vi "DEMPSubViewer.vi"() -> ()   [LabVIEW 2022 SP3]
panel:
  out "Channels":T1(array[cluster])
  out "bias":dbl[](array[numeric])
  out "times":dbl[](array[numeric])
  in  "Path":path
  in  "IV Phase":i64=-42
  out "XAxis":dbl[](array[numeric])
  in  "Channel Name":string
  in  "XChannel":bool
  in  "XBias":bool
  in  "XTime":bool
  out "Y Scale":i64
  in  "10 nA":bool
  in  "5nA":bool
  in  "3nA":bool
  in  "1nA":bool
  in  "Y Limits":bool
  out "XY Graph 32":cluster{dbl[], "Data":dbl[]}[](graph)
  out "XY Graph 31":cluster{dbl[], "Data":dbl[]}[](graph)
  out "XY Graph 30":cluster{dbl[], "Data":dbl[]}[](graph)
  out "XY Graph 29":cluster{dbl[], "Data":dbl[]}[](graph)
  out "XY Graph 28":cluster{dbl[], "Data":dbl[]}[](graph)
  out "XY Graph 27":cluster{dbl[], "Data":dbl[]}[](graph)
  out "XY Graph 26":cluster{dbl[], "Data":dbl[]}[](graph)
  out "XY Graph 25":cluster{dbl[], "Data":dbl[]}[](graph)
  out "XY Graph 24":cluster{dbl[], "Data":dbl[]}[](graph)
  out "XY Graph 23":cluster{dbl[], "Data":dbl[]}[](graph)
  out "XY Graph 22":cluster{dbl[], "Data":dbl[]}[](graph)
  out "XY Graph 21":cluster{dbl[], "Data":dbl[]}[](graph)
  out "XY Graph 20":cluster{dbl[], "Data":dbl[]}[](graph)
  out "XY Graph 19":cluster{dbl[], "Data":dbl[]}[](graph)
  out "XY Graph 18":cluster{dbl[], "Data":dbl[]}[](graph)
  out "XY Graph 17":cluster{dbl[], "Data":dbl[]}[](graph)
  out "XY Graph 16":cluster{dbl[], "Data":dbl[]}[](graph)
  out "XY Graph 15":cluster{dbl[], "Data":dbl[]}[](graph)
  out "XY Graph 14":cluster{dbl[], "Data":dbl[]}[](graph)
  out "XY Graph 13":cluster{dbl[], "Data":dbl[]}[](graph)
  out "XY Graph 12":cluster{dbl[], "Data":dbl[]}[](graph)
  out "XY Graph 11":cluster{dbl[], "Data":dbl[]}[](graph)
  out "XY Graph 10":cluster{dbl[], "Data":dbl[]}[](graph)
  out "XY Graph 9":cluster{dbl[], "Data":dbl[]}[](graph)
  out "XY Graph 3":cluster{dbl[], "Data":dbl[]}[](graph)
  out "XY Graph 8":cluster{dbl[], "Data":dbl[]}[](graph)
  out "XY Graph 7":cluster{dbl[], "Data":dbl[]}[](graph)
  out "XY Graph 6":cluster{dbl[], "Data":dbl[]}[](graph)
  out "XY Graph 5":cluster{dbl[], "Data":dbl[]}[](graph)
  out "XY Graph 4":cluster{dbl[], "Data":dbl[]}[](graph)
  out "XY Graph 2":cluster{dbl[], "Data":dbl[]}[](graph)
  out "XY Graph 1":cluster{dbl[], "Data":dbl[]}[](graph)
  in  "stop":bool
  # "X Axis"
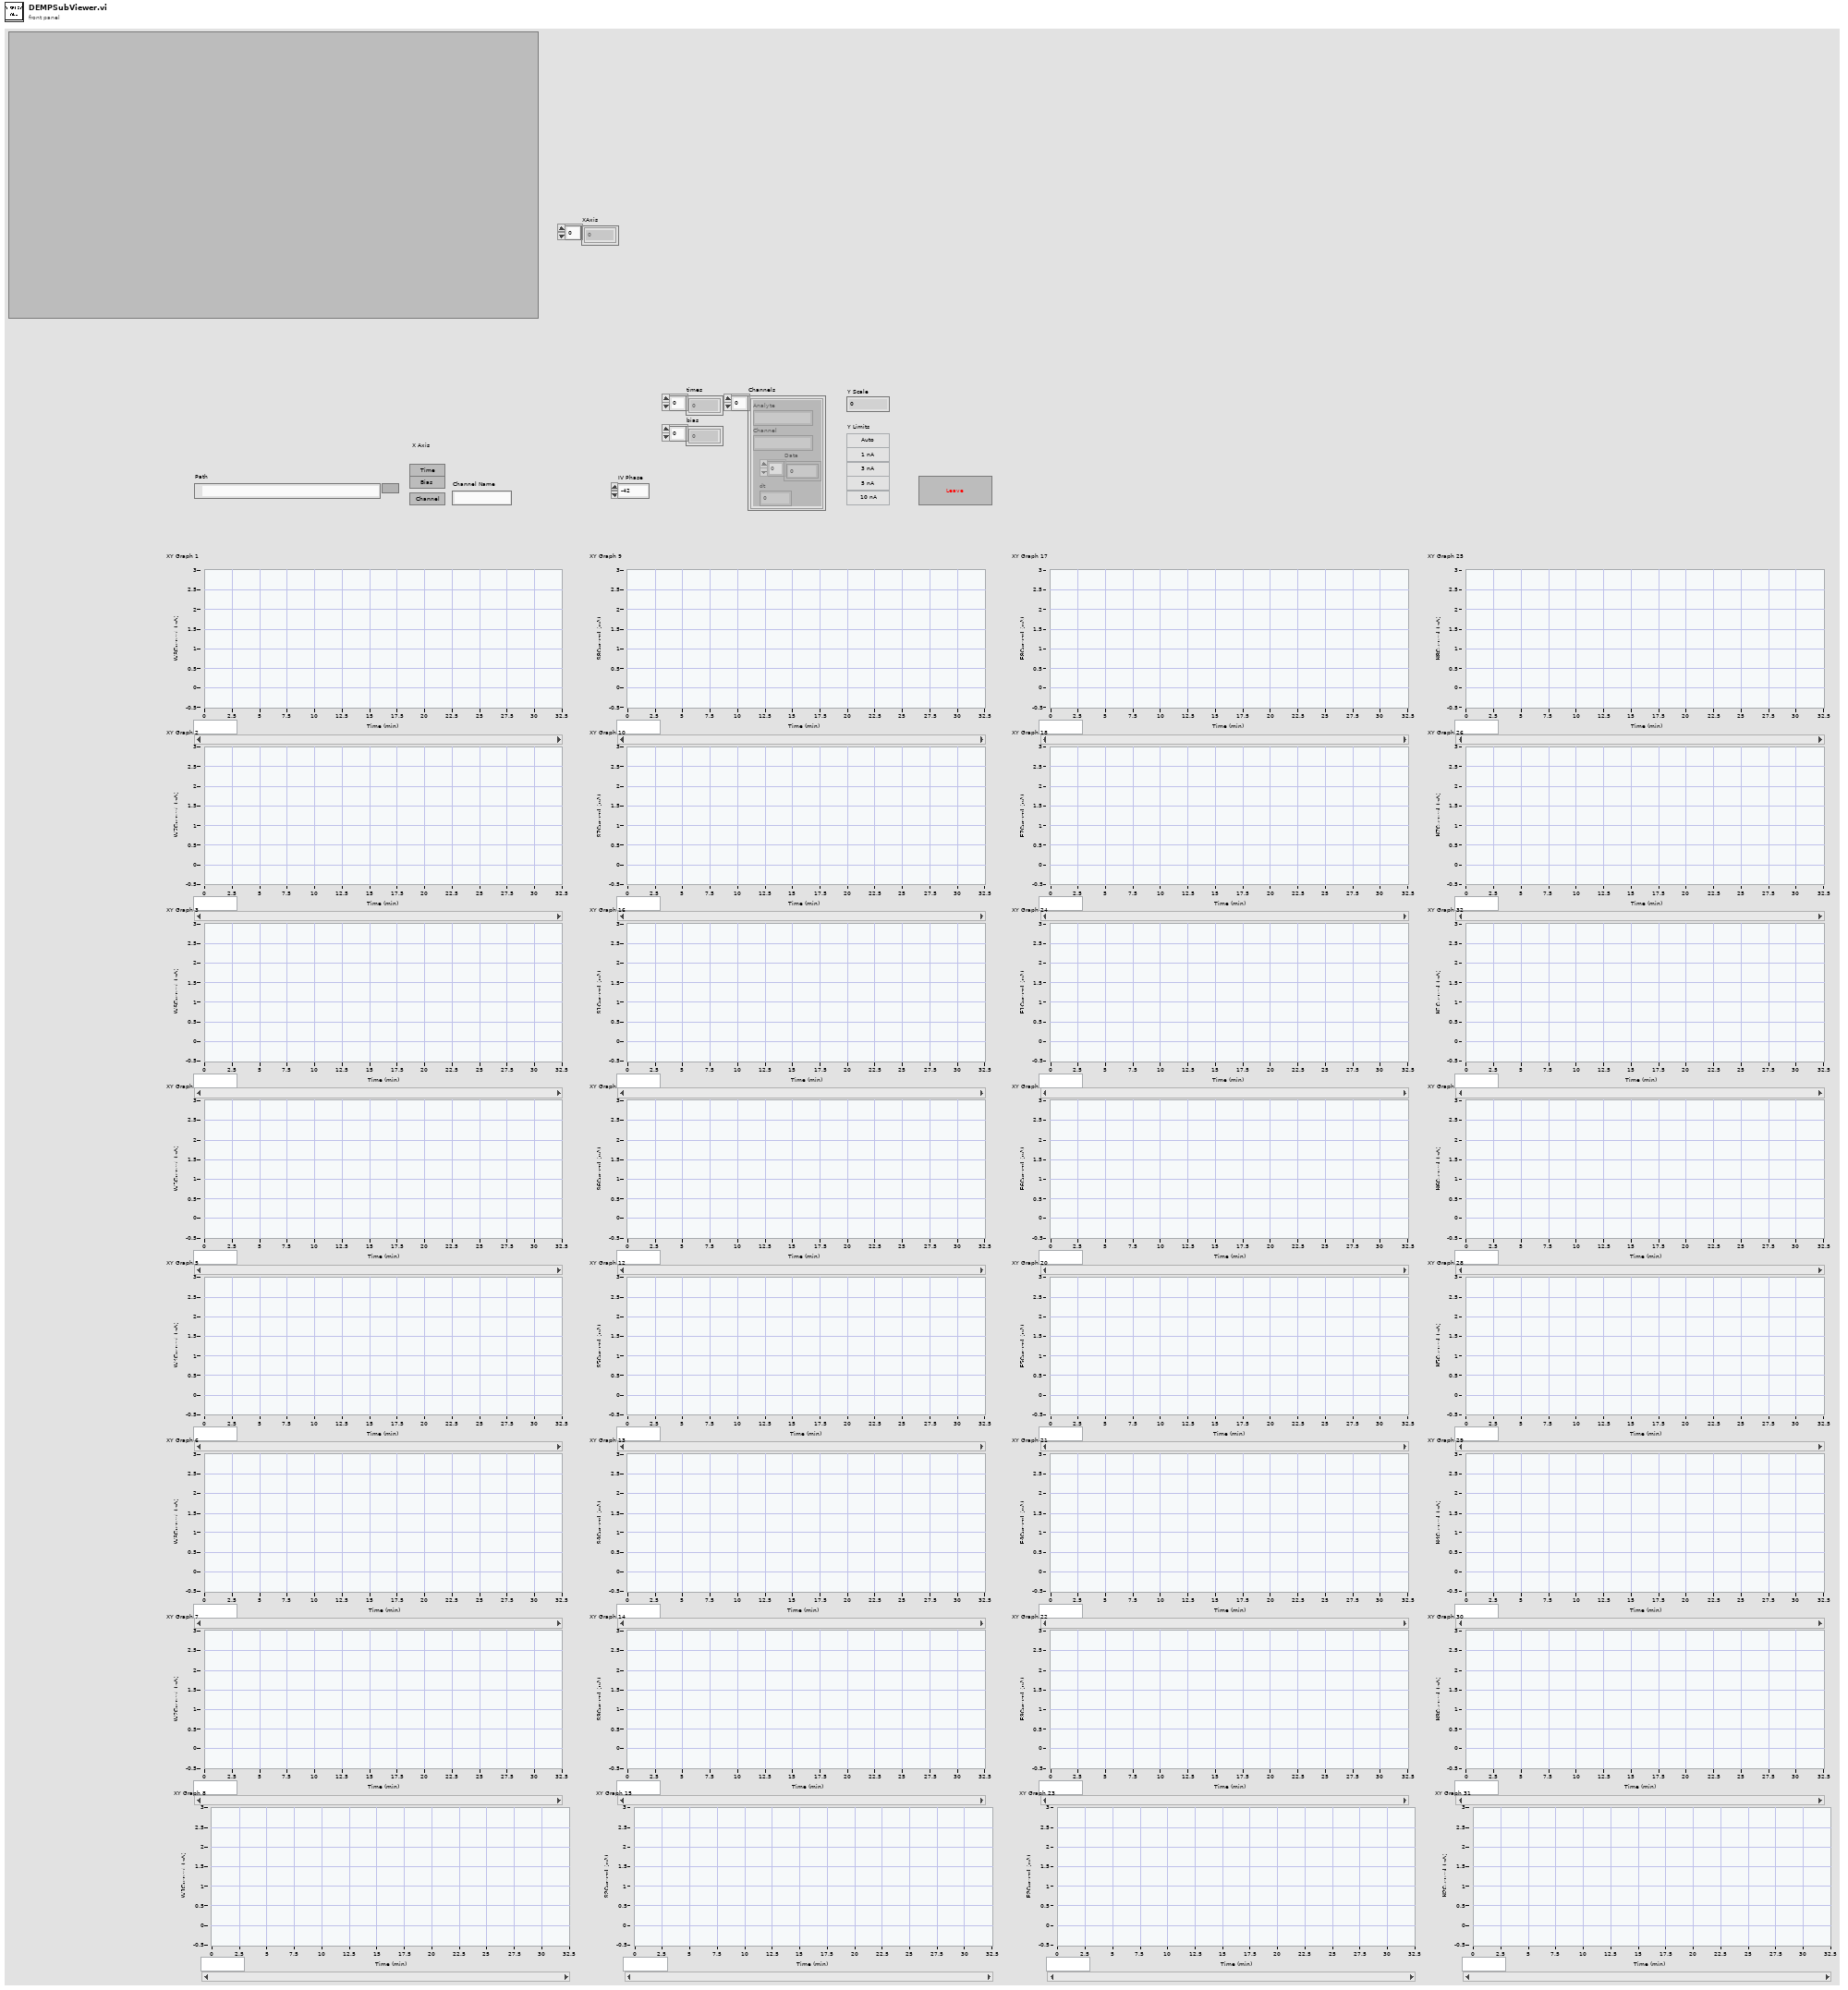
[diagram p1: front panel]
types:
  T1 = cluster{"Analyte":string, "Channel":string, "Data":dbl[], "dt":dbl}[]
  T2 = cluster{"Analyte":string, "Channel":string, "Data":dbl[], "dt":dbl}
  T3 = enum16{"open", "open or create", "create or replace", "create", "open (read-only)"}
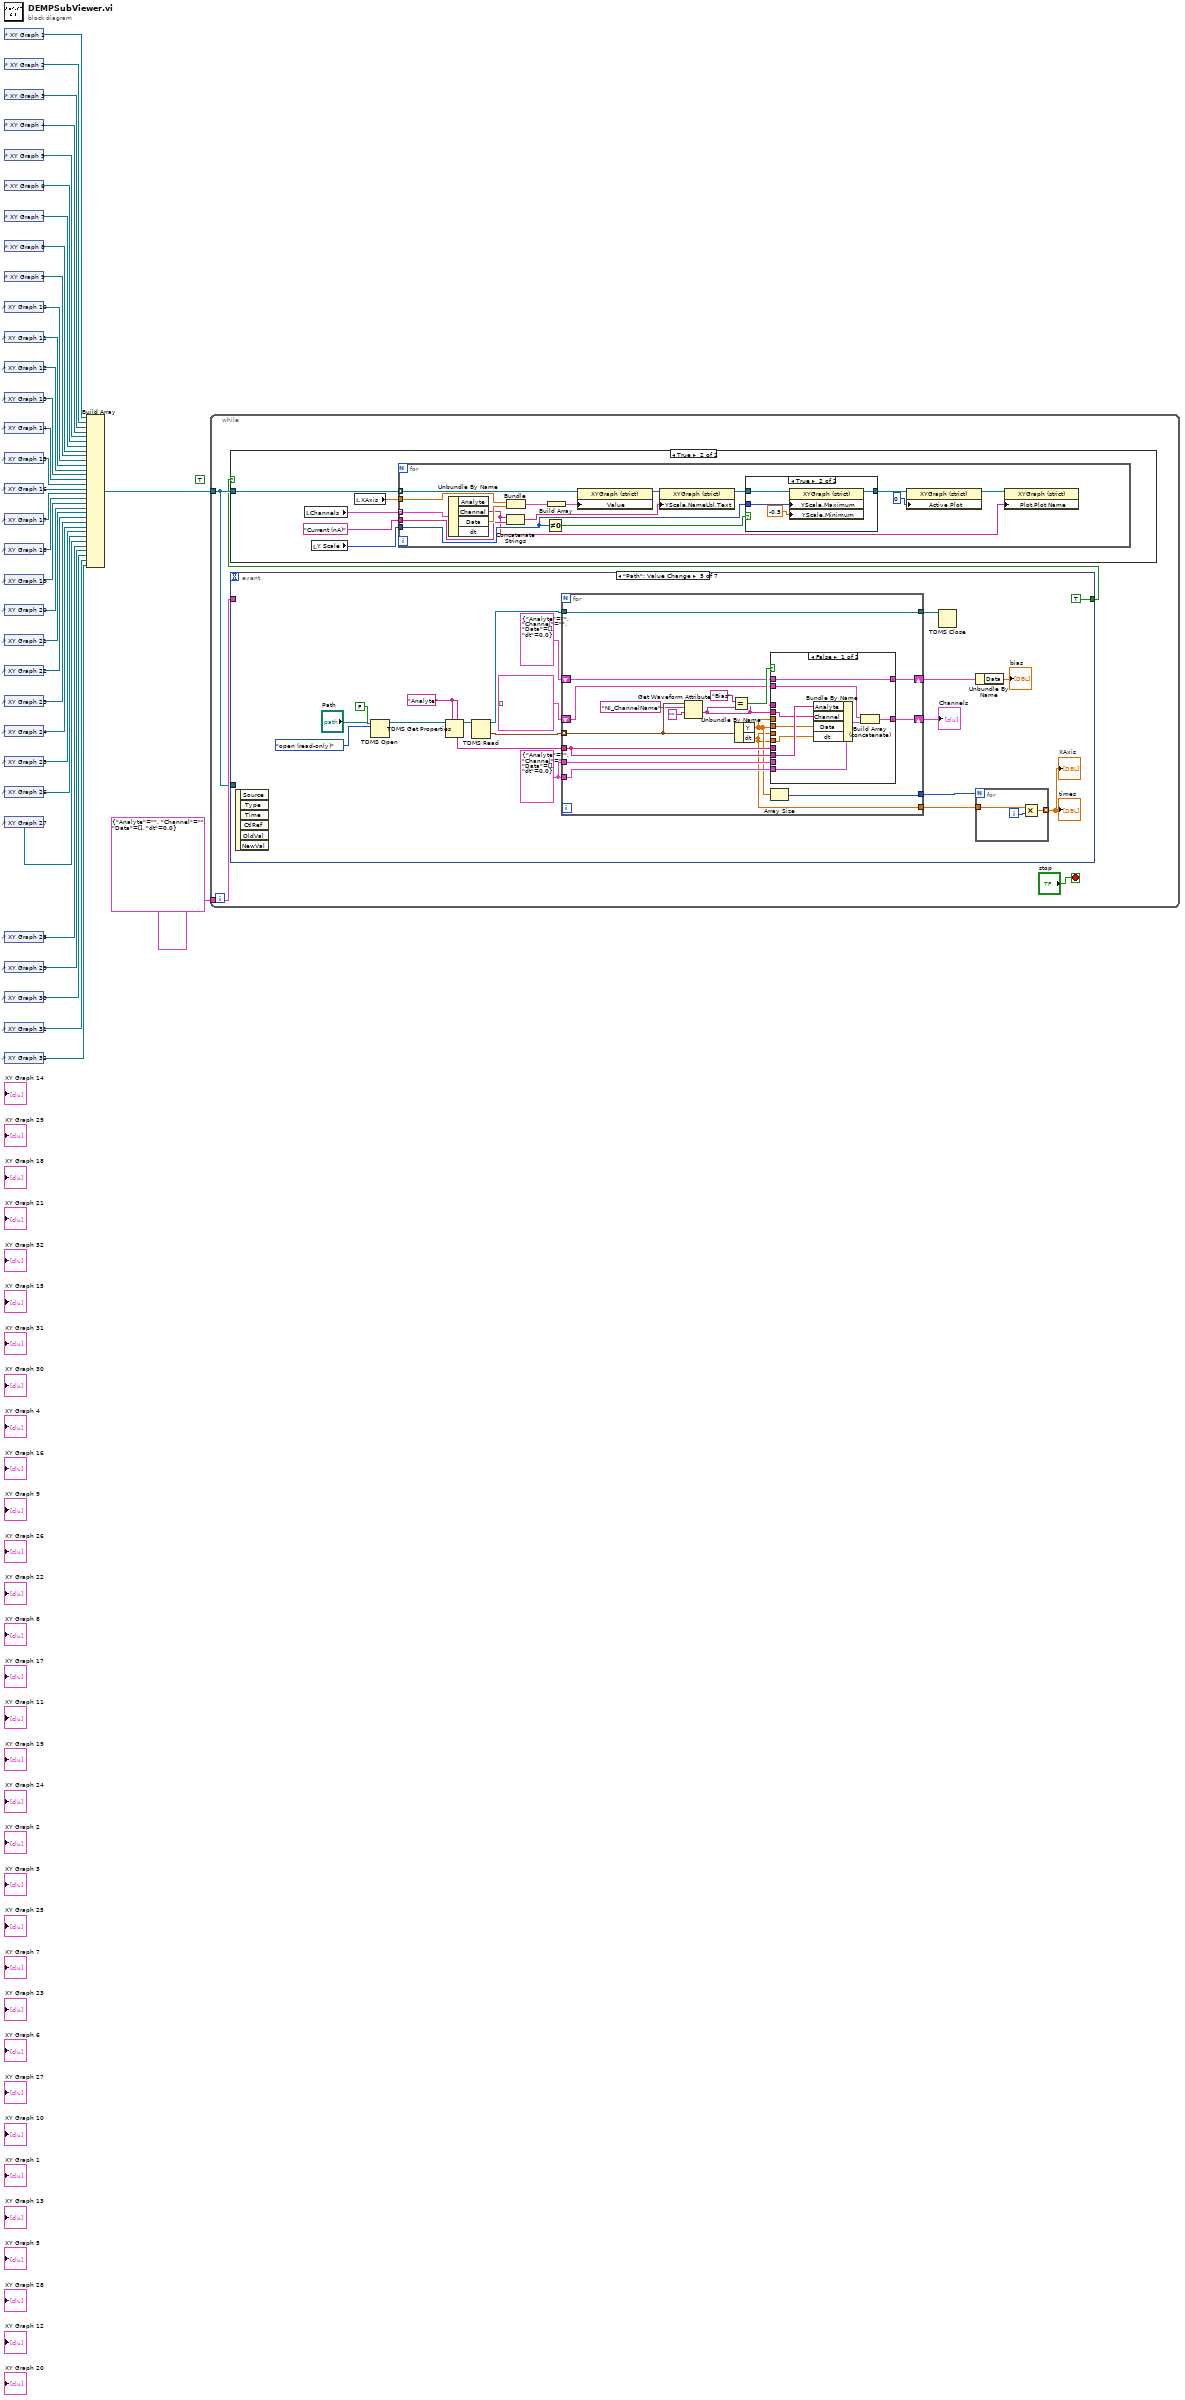
[diagram p0: block diagram]
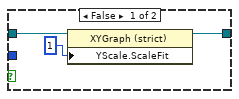
[diagram p3: hidden frame]
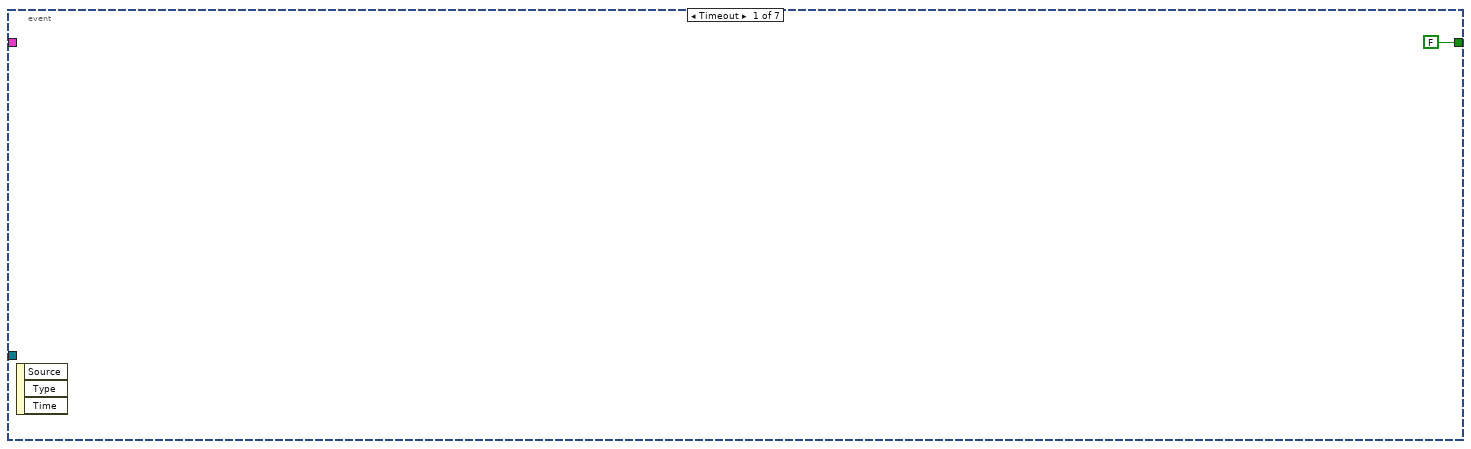
[diagram p4: hidden frame]
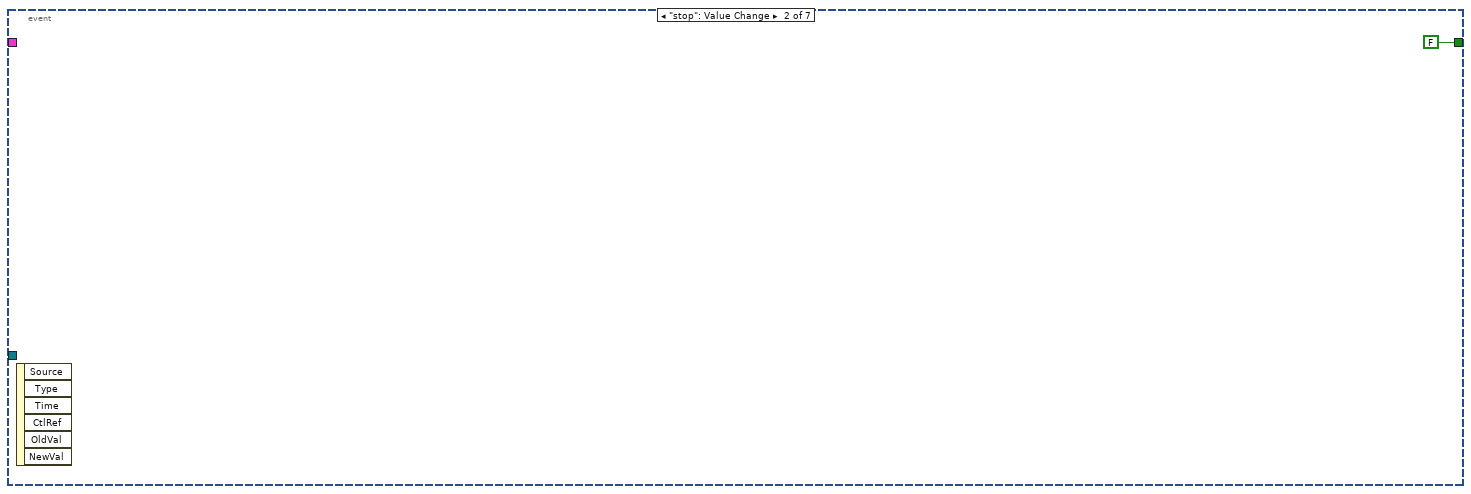
[diagram p5: hidden frame]
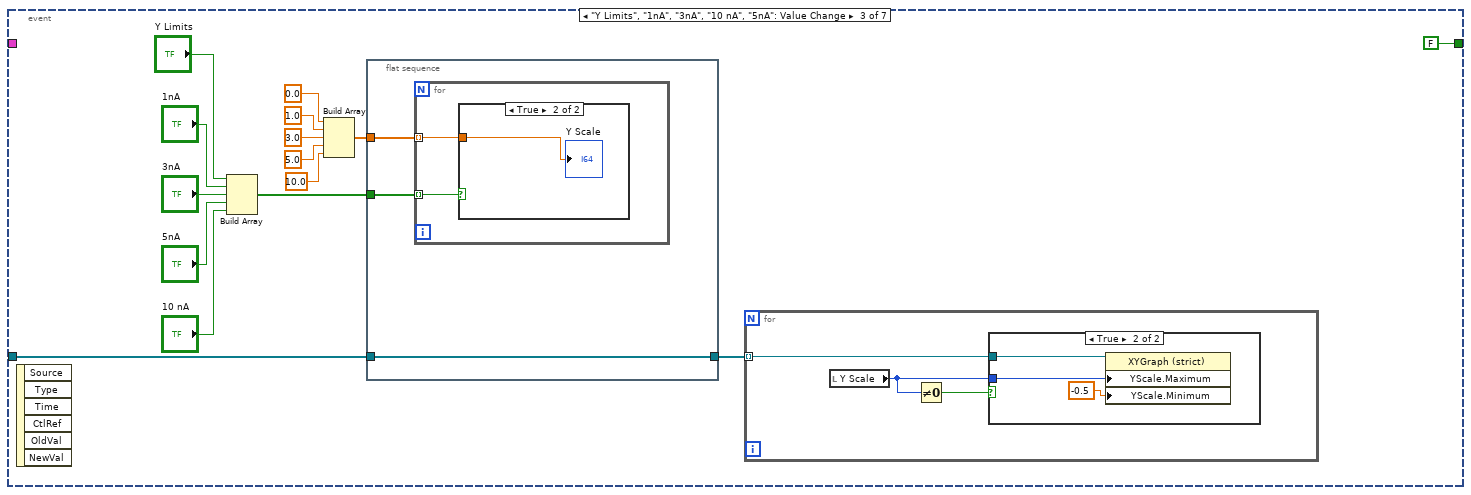
[diagram p6: hidden frame]
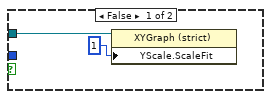
[diagram p8: hidden frame]
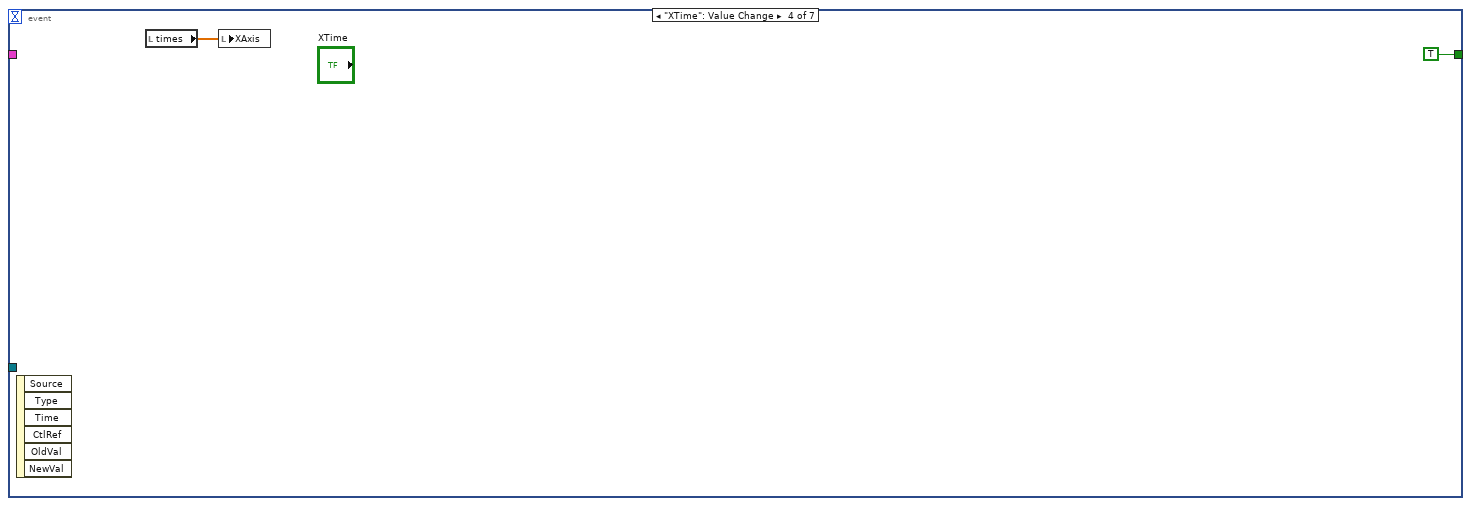
[diagram p9: hidden frame]
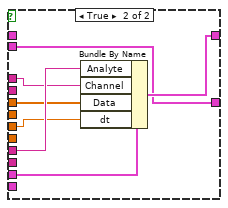
[diagram p10: hidden frame]
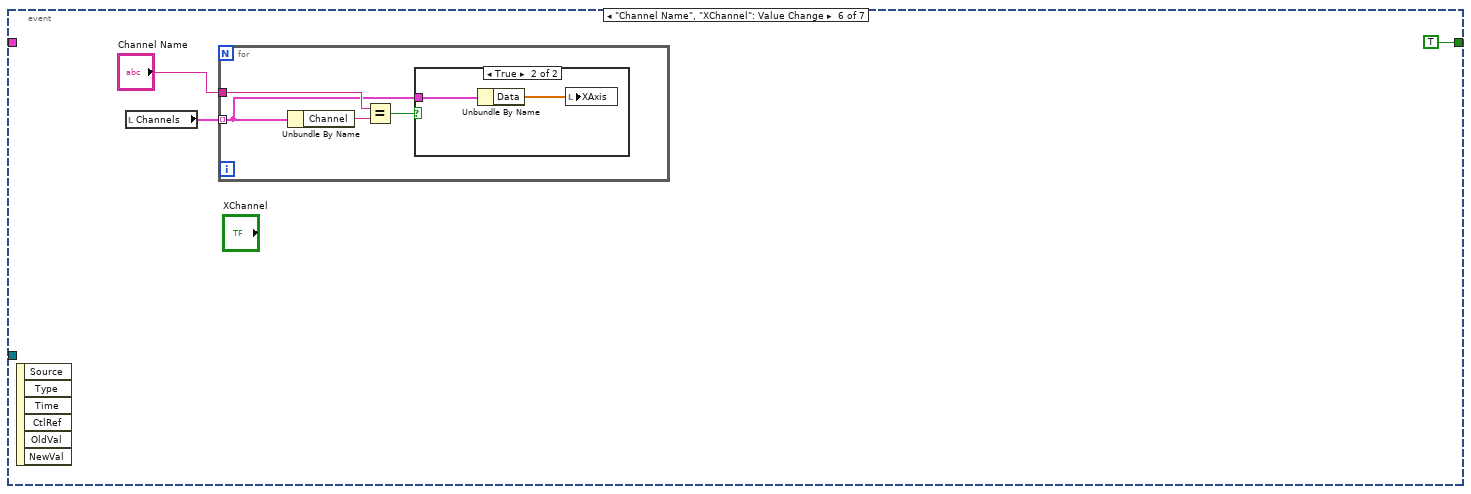
[diagram p11: hidden frame]
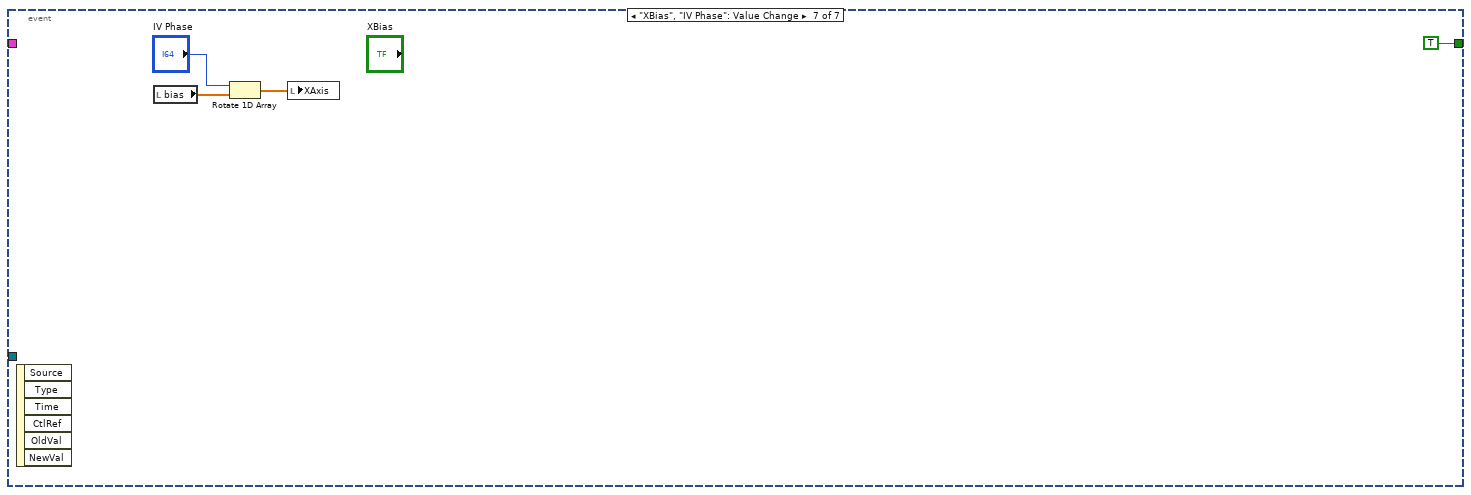
[diagram p13: hidden frame]
diagram:
  (unwired) TRUE
  n1 = control-ref of="XY Graph 1"() -> (w33:refnum<vi>)
  n2 = control-ref of="XY Graph 2"() -> (w32:refnum<vi>)
  n3 = control-ref of="XY Graph 3"() -> (w31:refnum<vi>)
  n4 = control-ref of="XY Graph 4"() -> (w30:refnum<vi>)
  n5 = control-ref of="XY Graph 5"() -> (w29:refnum<vi>)
  n6 = control-ref of="XY Graph 6"() -> (w28:refnum<vi>)
  n7 = control-ref of="XY Graph 7"() -> (w27:refnum<vi>)
  n8 = control-ref of="XY Graph 8"() -> (w26:refnum<vi>)
  n9 = control-ref of="XY Graph 9"() -> (w25:refnum<vi>)
  n10 = control-ref of="XY Graph 10"() -> (w24:refnum<vi>)
  n11 = control-ref of="XY Graph 11"() -> (w23:refnum<vi>)
  n12 = control-ref of="XY Graph 12"() -> (w22:refnum<vi>)
  n13 = control-ref of="XY Graph 13"() -> (w21:refnum<vi>)
  n14 = control-ref of="XY Graph 14"() -> (w20:refnum<vi>)
  n15 = control-ref of="XY Graph 15"() -> (w19:refnum<vi>)
  n16 = control-ref of="XY Graph 16"() -> (w18:refnum<vi>)
  n17 = control-ref of="XY Graph 17"() -> (w17:refnum<vi>)
  n18 = control-ref of="XY Graph 18"() -> (w16:refnum<vi>)
  n19 = control-ref of="XY Graph 19"() -> (w15:refnum<vi>)
  n20 = control-ref of="XY Graph 20"() -> (w14:refnum<vi>)
  n21 = control-ref of="XY Graph 21"() -> (w13:refnum<vi>)
  n22 = control-ref of="XY Graph 22"() -> (w12:refnum<vi>)
  n23 = control-ref of="XY Graph 23"() -> (w11:refnum<vi>)
  n24 = control-ref of="XY Graph 24"() -> (w10:refnum<vi>)
  n25 = control-ref of="XY Graph 25"() -> (w9:refnum<vi>)
  n26 = control-ref of="XY Graph 26"() -> (w8:refnum<vi>)
  n27 = control-ref of="XY Graph 27"() -> (w7:refnum<vi>)
  n28 = control-ref of="XY Graph 28"() -> (w6:refnum<vi>)
  n29 = control-ref of="XY Graph 29"() -> (w5:refnum<vi>)
  n30 = control-ref of="XY Graph 30"() -> (w4:refnum<vi>)
  n31 = control-ref of="XY Graph 31"() -> (w3:refnum<vi>)
  n32 = control-ref of="XY Graph 32"() -> (w2:refnum<vi>)
  n33 = Build Array(w33, w32, w31, w30, w29, w28, w27, w26, w25, w24, w23, w22, w21, w20, w19, w18, w17, w16, w15, w14, w13, w12, w11, w10, w9, w8, w7, w6, w5, w4, w3, w2) -> (w1:refnum<vi>[])
  n34 = while {
    tunnel: T2 {"Analyte"="", "Channel"="", "Data"=[], "dt"=0.0} -> [w37]
    tunnel: w1 -> [w36]
    stop <- "stop" stop-if-true
    n35 = event shown="[4] \"Path\": Value Change" {
      selector: _ -> [_ _ _ _ _ _ _]
      dyn-events: _ -> [_ _ _ _ _ _ _]
      timeout: _ -> [_ _ _ _ _ _ _]
      tunnel: w37 -> [_ _ _ _ _ _ _]
      tunnel: [FALSE FALSE FALSE TRUE TRUE TRUE TRUE] -> w35
      tunnel: w36 -> [_ _ w69 _ _ _ _]
      event Timeout {
        n36 = event-data() -> ()  [unwired: 1 in, 3 out]
      }
      event "stop": Value Change {
        n37 = event-data() -> ()  [unwired: 1 in, 6 out]
      }
      event "Y Limits", "1nA", "3nA", "10 nA", "5nA": Value Change {
        n38 = event-data() -> ()  [unwired: 1 in, 6 out]
        n39 = Build Array("Y Limits", "1nA", "3nA", "5nA", "10 nA") -> (w83:bool[])
        n40 = Build Array(0.0 ("element"), 1.0 ("element"), 3.0 ("element"), 5.0 ("element"), 10.0 ("element")) -> (w82:dbl[])
        n41 = flat-sequence {
          tunnel: w83 -> [w86]
          tunnel: w82 -> [w85]
          tunnel: [w84] -> w70
          tunnel: w69 -> [w84]
          frame #0 {
            n42 = for {
              tunnel: w86 -> [w88] mode=indexing
              tunnel: w85 -> [w87] mode=indexing
              n43 = case shown="True" w88 {
                tunnel: w87 -> [_ w89]
                frame False {
                }
                frame True {
                  "Y Scale" <- w89
                }
              }
            }
          }
        }
        n44 = for {
          tunnel: w70 -> [w90] mode=indexing
          n45 = local read "Y Scale"() -> (w91:i64)
          n46 = Not Equal To 0?(x=w91) -> (x != 0?=w92:bool)
          n47 = case shown="True" w92 {
            tunnel: w90 -> [w94 w97]
            tunnel: w91 -> [_ w96]
            frame False {
              n48 = property on="Property Node" class="XYGraph (strict)"(reference=w94, "YScale.ScaleFit"=u8 1 ("Y Scale.Scale Fit")) -> ()  [unwired: 1 in, 2 out]
            }
            frame True {
              n49 = property on="Property Node" class="XYGraph (strict)"(reference=w97, "YScale.Maximum"=w96, "YScale.Minimum"=-0.5 ("X Scale.Range:Minimum")) -> ()  [unwired: 1 in, 2 out]
            }
          }
        }
      }
      event "XTime": Value Change {
        n50 = event-data() -> ()  [unwired: 1 in, 6 out]
        n51 = local read "times"() -> (w98:dbl[])
        n52 = local write "XAxis"(w98) -> ()
      }
      event "Path": Value Change {
        w116 = "Analyte"
        w118 = T2 {"Analyte"="", "Channel"="", "Data"=[], "dt"=0.0} ("element")
        n53 = event-data() -> ()  [unwired: 1 in, 6 out]
        n54 = TDMS Open(5:FALSE ("create index file? (T)"), 10:T3."open (read-only)" ("operation (0:open)"), 11:"Path") -> (3:w112:refnum<k34>)  [unwired: 4 in, 1 out]
        n55 = TDMS Get Properties(5:w116, 7:w116, 11:w112) -> (3:w115:refnum<k34>, 4:w113:string)  [unwired: 3 in, 4 out]
        n56 = TDMS Read(0:w115) -> (4:w111:refnum<k34>, 10:w114:waveform(dbl)[])  [unwired: 7 in, 4 out]
        n57 = for {
          tunnel: w114 -> [w139] mode=indexing
          tunnel: w113 -> [w129]
          tunnel: [w136] -> w110
          tunnel: w111 -> [w136]
          tunnel: w118 -> [w130]
          tunnel: w118 -> [w133]
          shift-right: [w132] -> w119
          shift-left: T2 {"Analyte"="", "Channel"="", "Data"=[], "dt"=0.0} ("element") -> [w131]
          shift-right: [w127] -> w102
          shift-left: T1 [] -> [w126]
          tunnel: [w124] -> w107
          tunnel: [w123] -> w106
          n58 = Get Waveform Attribute(5:"", 6:"NI_ChannelName" ("name"), 7:w139) -> (1:w128:string)  [unwired: 1 in, 3 out]
          n59 = Equal?(x="Bias", y=w128) -> (x = y?=w134:bool)
          n60 = Unbundle By Name(w139) -> ("Y"=w125:dbl[], "dt"=w123:dbl)
          n61 = case shown="False" w134 {
            tunnel: w129 -> [_ w155]
            tunnel: w128 -> [_ w154]
            tunnel: w125 -> [_ w153]
            tunnel: w123 -> [_ w152]
            tunnel: w133 -> [_ w151]
            tunnel: [w148 w150] -> w132
            tunnel: w131 -> [w148 _]
            tunnel: w130 -> [w147 _]
            tunnel: w129 -> [w146 _]
            tunnel: w128 -> [w145 _]
            tunnel: w125 -> [w144 _]
            tunnel: w123 -> [w143 _]
            tunnel: [w142 w149] -> w127
            tunnel: w126 -> [w140 w149]
            frame False {
              n62 = Bundle By Name(cluster=w147, "Analyte"=w146, "Channel"=w145, "Data"=w144, "dt"=w143) -> (w141:T2)
              n63 = Build Array (concatenate)(w140, w141) -> (w142:T1)
            }
            frame True {
              n64 = Bundle By Name(cluster=w151, "Analyte"=w155, "Channel"=w154, "Data"=w153, "dt"=w152) -> (w150:T2)
            }
          }
          n65 = Array Size(array=w125) -> (size(s)=w124:i32)
        }
        "Channels" <- w102
        n66 = TDMS Close(11:w110) -> ()  [unwired: 1 in, 2 out]
        n67 = Unbundle By Name(w119) -> ("Data"=→"bias":dbl[])
        n68 = for {
          N: w107 -> [_]
          tunnel: w106 -> [w122]
          tunnel: [w120] -> w105 mode=indexing
          i -> [w121]
          n69 = Multiply(x=w122, y=w121) -> (x*y=w120:dbl)
        }
        "XAxis" <- w105
        "times" <- w105
      }
      event "Channel Name", "XChannel": Value Change {
        n70 = event-data() -> ()  [unwired: 1 in, 6 out]
        n71 = local read "Channels"() -> (w156:T1)
        n72 = for {
          tunnel: "Channel Name" -> [w161]
          tunnel: w156 -> [w159] mode=indexing
          n73 = Unbundle By Name(w159) -> ("Channel"=w162:string)
          n74 = Equal?(x=w161, y=w162) -> (x = y?=w160:bool)
          n75 = case shown="True" w160 {
            tunnel: w159 -> [_ w163]
            frame False {
            }
            frame True {
              n76 = Unbundle By Name(w163) -> ("Data"=w164:dbl[])
              n77 = local write "XAxis"(w164) -> ()
            }
          }
        }
      }
      event "XBias", "IV Phase": Value Change {
        n78 = event-data() -> ()  [unwired: 1 in, 6 out]
        n79 = local read "bias"() -> (w165:dbl[])
        n80 = Rotate 1D Array(1:w165, 2:"IV Phase") -> (0:w166:dbl[])
        n81 = local write "XAxis"(w166) -> ()
      }
    }
    n82 = case shown="True" w35 {
      tunnel: w36 -> [_ w43]
      frame False {
      }
      frame True {
        n83 = local read "Channels"() -> (w39:T1)
        n84 = local read "Y Scale"() -> (w42:i64)
        n85 = local read "XAxis"() -> (w40:dbl[])
        n86 = for {
          tunnel: w43 -> [w44] mode=indexing
          tunnel: w42 -> [w59]
          tunnel: "Current (nA)" -> [w51]
          tunnel: w40 -> [w48]
          tunnel: w39 -> [w45] mode=indexing
          n87 = Unbundle By Name(w45) -> ("Channel"=w46:string, "Data"=w54:dbl[])  [unwired: 2 out]
          n88 = Concatenate Strings(w46, w51) -> (w47:string)
          n89 = Bundle("XAxis"=w48, "Data"=w54) -> (w53:cluster{"XAxis":dbl[], "Data":dbl[]})  [unwired: 1 in]
          n90 = Not Equal To 0?(x=w59) -> (x != 0?=w58:bool)
          n91 = Build Array(w53) -> (w52:cluster{"XAxis":dbl[], "Data":dbl[]}[])
          n92 = property on="Property Node" class="XYGraph (strict)"(reference=w44, "Value"=w52) -> (reference out=w57:refnum<vi>)  [unwired: 1 in, 1 out]
          n93 = property on="Property Node" class="XYGraph (strict)"(reference=w57, "YScale.NameLbl.Text"=w47) -> (reference out=w56:refnum<vi>)  [unwired: 1 in, 1 out]
          n94 = case shown="True" w58 {
            tunnel: w56 -> [w62 w66]
            tunnel: w59 -> [_ w65]
            tunnel: [w60 w63] -> w55
            frame False {
              n95 = property on="Property Node" class="XYGraph (strict)"(reference=w62, "YScale.ScaleFit"=u8 1 ("Y Scale.Scale Fit")) -> (reference out=w60:refnum<vi>)  [unwired: 1 in, 1 out]
            }
            frame True {
              n96 = property on="Property Node" class="XYGraph (strict)"(reference=w66, "YScale.Maximum"=w65, "YScale.Minimum"=-0.5 ("X Scale.Range:Minimum")) -> (reference out=w63:refnum<vi>)  [unwired: 1 in, 1 out]
            }
          }
          n97 = property on="Property Node" class="XYGraph (strict)"(reference=w55, "Active Plot"=u32 0) -> (reference out=w50:refnum<vi>)  [unwired: 1 in, 1 out]
          n98 = property on="Property Node" class="XYGraph (strict)"(reference=w50, "Plot.Plot Name"=w46) -> ()  [unwired: 1 in, 2 out]
        }
      }
    }
  }
